vi "Tmp_M simulated main.vi"(8 "Error In":errorcluster, 9 "timeout ms":i32=1000, 10 "Queue to master":T2, 11 "Module queue":T2) -> (0 "Error Out":errorcluster, 1 "Connected":bool=TRUE, 3 "Temperatures":T1[](array[typedef]) {"Time stamp" format="%<%H:%M:%S%2u\n%Y/%m/%d>T"})   [LabVIEW 2021, in "Magnet module.lvlib"]
doc: "Magnet module controls: power supply unit (PSU/SMS) and temperature monitor (TM/LSC218).\nPSU controls mainly: switch heater and ramping of current which runs throught coil.\nTM controls temperature of switch, coil and cryostat.\nMessage for magnet is a cluster that contains: {(enum) Command , (variant) Data}\nFor simplifieing of documentation, the Command is noted as a name of instruction, and Data is represented by a requered datatype (mostly cluster) name.\nCommands:\nInitialize(Magnet Config Constants) - Sugesstion: Load configuration constants from configuration file.\nSet field (Set field{B, R, cr}) - B-field[T], R-ramp[A/s], cr - custom ramp[bool].\nSwitch mode(mode) - to persistant, or to ramping.\nBlackout() - undone functionality of emergency deenergizing.\nUpdate() - Important! This triggers update of data from instruments. Shoud occure in regular intervals as priority message.\nResponses:\nMagnet initialized ();\nTM revision(temperature monitor revision);\nMagnet init error(error);\nSetting field(Set Field{B, R, cr});\nWarning(string);\nSwitching to(mode);\nUpdate error(error);\nTM update(TM sensors);\nPSU update(PSU data);\nMagnet status();"
uses:
  Magnet module.lvlib
  ctl/Cryostat temperature sensors.ctl
  Messenger service/Data types/Module name.ctl
  Messenger service/MessengerLib.lvlib
  submodules/Temperature monitor/Temperature monitor.lvlib
  Messenger service/Data types/Mailbox address.ctl
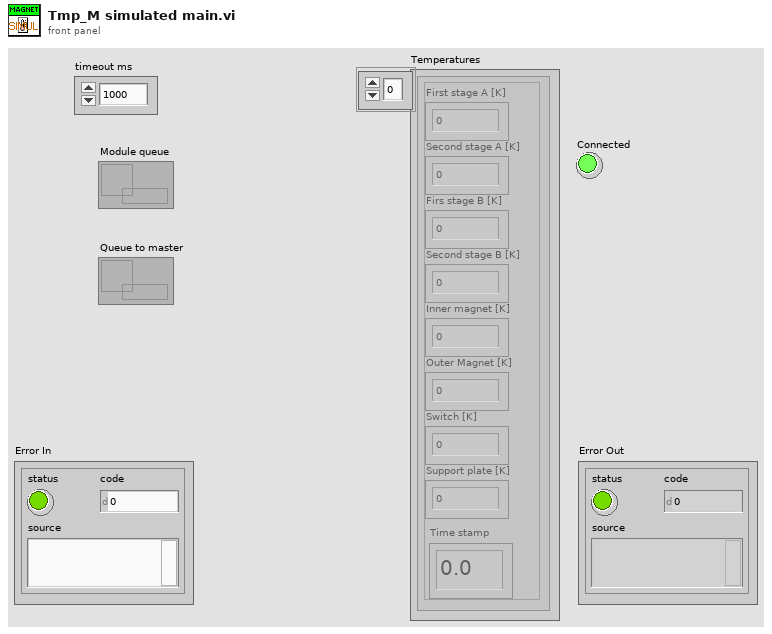
[diagram p1: front panel]
types:
  T1 = typedef "Cryostat temperature sensors.ctl" = cluster{"First stage A [K]":dbl, "Second stage A [K]":dbl, "Firs stage B [K]":dbl, "Second stage B [K]":dbl, "Inner magnet [K]":dbl, "Outer Magnet [K]":dbl, "Switch [K]":dbl, "Support plate [K]":dbl, "Time stamp":dbl}
  T2 = typedef "MessengerLib.lvlib/Mailbox address.ctl" = refnum<queue>
  T3 = typedef "MessengerLib.lvlib/Module name.ctl" = enum16{"Emty", "Magnet", "VTI", "Excitation", "Servo", "Acquisition", "Rotator", "Digitizer", "SMU2450", "Carousel", "Multimeter", "Tmp monitor", "Power monitor"}
  T4 = typedef "Temperature monitor.lvlib/Tmp_M commands.ctl" = enum16{"Ignore", "Log", "Connect", "Set timeout", "Update", "Disconnect", "End"}
  T5 = typedef "Temperature monitor.lvlib/TM Revision.ctl" = cluster{"Instr Serial Number":string, "Instr Driver Revision":string, "Instr Firmware Revision":string, "Instr Model Number":string}
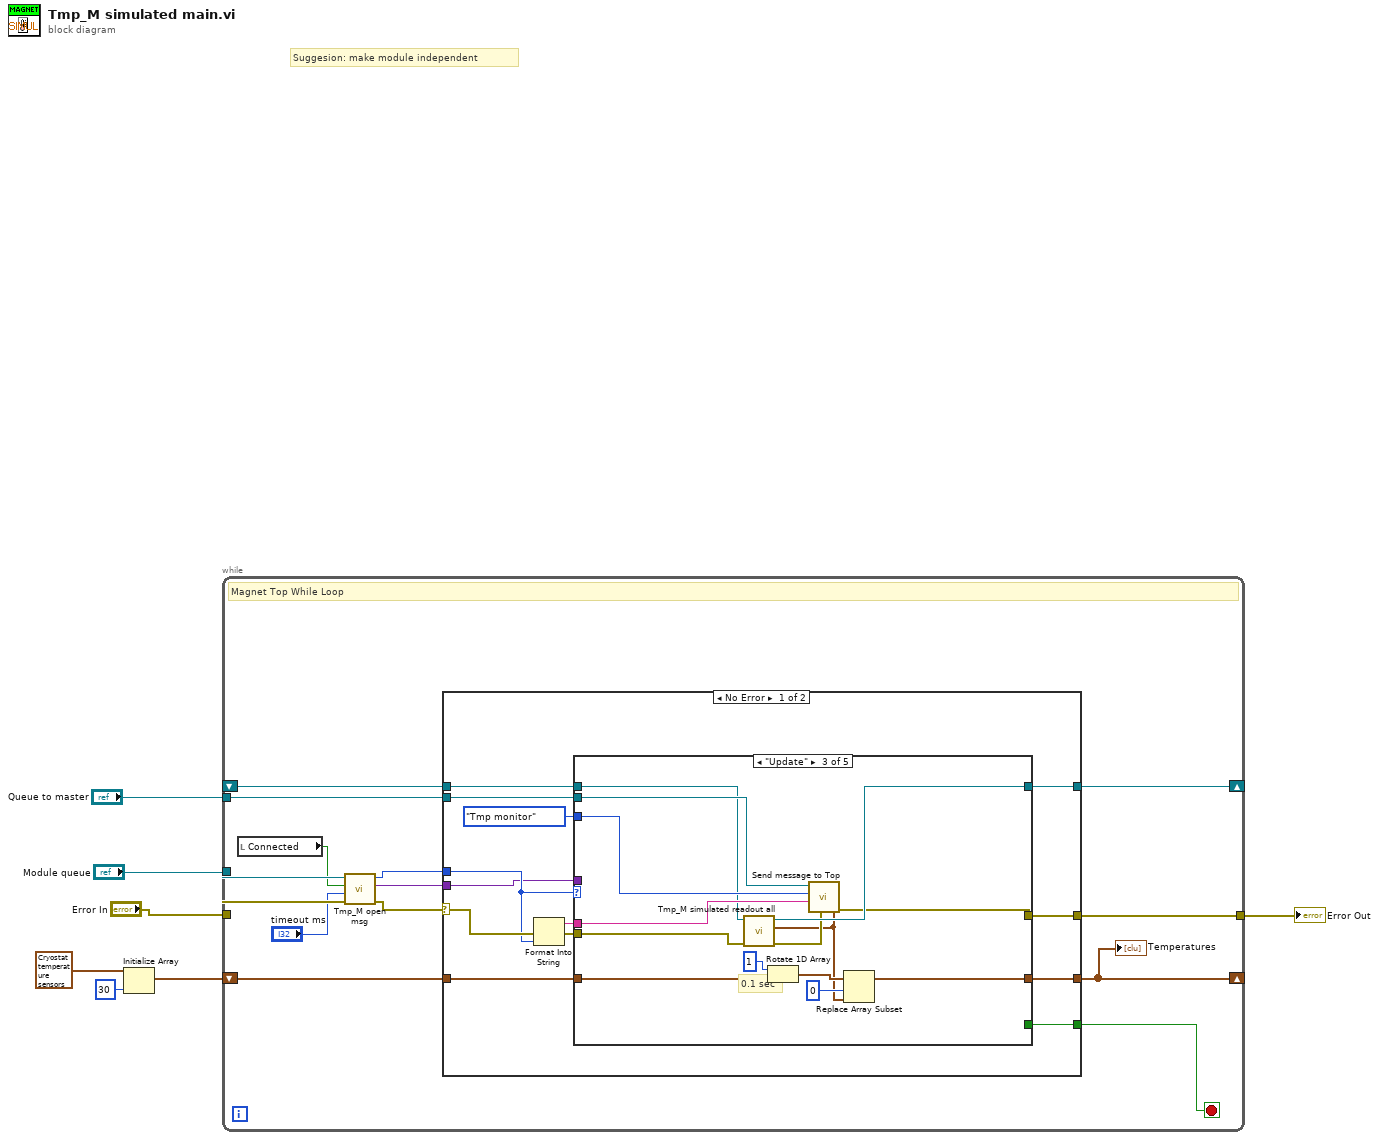
[diagram p0: block diagram]
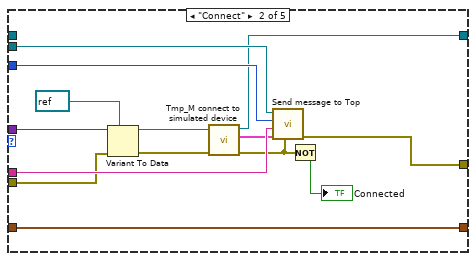
[diagram p3: hidden frame]
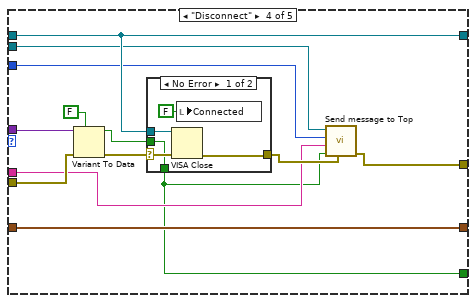
[diagram p4: hidden frame]
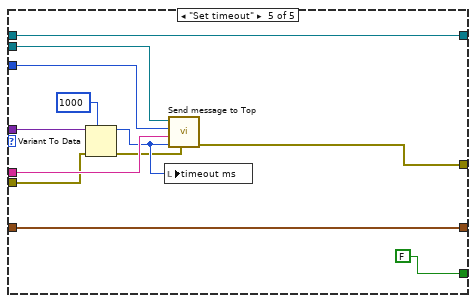
[diagram p6: hidden frame]
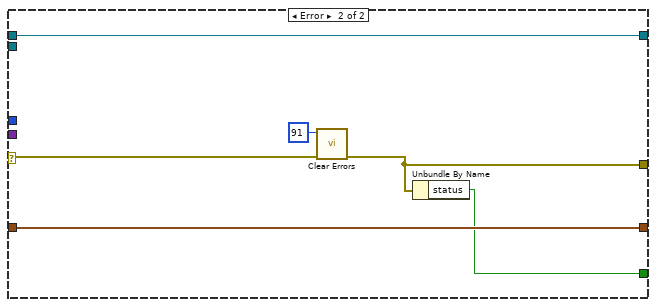
[diagram p7: hidden frame]
diagram:
  # "Suggesion: make module independent"
  n1 = Initialize Array(T1 {"First stage A [K]"=0.0, "Second stage A [K]"=0.0, "Firs stage B [K]"=0.0, "Second stage B [K]"=0.0, "Inner magnet [K]"=0.0, "Outer Magnet [K]"=0.0, "Switch [K]"=0.0, "Support plate [K]"=0.0, "Time stamp"=0.0} ("LSC218 sensors"), 30 ("dimension size")) -> (w5:T1[])
  n2 = while {
    tunnel: "Module queue" -> [w16]
    tunnel: "Queue to master" -> [w21]
    shift-right: [w19] -> _
    shift-left: w5 -> [w20]
    shift-right: [w18] -> _
    shift-left: _ -> [w17]
    tunnel: "Error In" -> [w15]
    tunnel: [w10] -> w1
    stop <- w9 stop-if-true
    # "Magnet Top While Loop"
    n3 = local read "Connected"() -> (w8:bool)
    n4 = call "Tmp_M open msg.vi"("error in (no error)"=w15, "timeout ms (1000)"="timeout ms", "Connected"=w8, "Queue in"=w16) -> ("error out"=w12:errorcluster, "Data"=w11:variant, "Command"=w14:T4)  [unwired: 3 in, 2 out]
    n5 = case shown="No Error" w12 {
      selector: w12 -> [w26 w101]
      tunnel: w21 -> [w34 _]
      tunnel: w14 -> [w25 _]
      tunnel: w20 -> [w33 w102]
      tunnel: [w32 w102] -> w19
      tunnel: [w22 w98] -> w9
      tunnel: [w29 w97] -> w18
      tunnel: w17 -> [w28 w97]
      tunnel: w11 -> [w24 _]
      tunnel: [w23 w99] -> w10
      frame No Error {
        n6 = Format Into String(error in=w26, w25) -> (resulting string=w30:string, error out=w27:errorcluster)  [unwired: 2 in]
        n7 = case shown="\"Update\"" w25 {
          tunnel: w34 -> [_ w51 w61 w70 w95]
          tunnel: w33 -> [w37 w50 w65 w78 w96]
          tunnel: [w37 w50 w64 w78 w96] -> w32
          tunnel: Module_name."Tmp monitor" ("Module") -> [_ w48 w62 w69 w92]
          tunnel: w30 -> [_ w49 w63 w68 w93]
          tunnel: [_ _ _ w66 FALSE] -> w22
          tunnel: [w36 w46 w59 w77 w91] -> w29
          tunnel: w28 -> [w36 _ w60 w77 w91]
          tunnel: w27 -> [w35 w42 w57 w74 w88]
          tunnel: w24 -> [_ w41 _ w75 w89]
          tunnel: [w35 w40 w58 w71 w85] -> w23
          frame "Ignore", Default {
          }
          frame "Connect" {
            n8 = Variant To Data(error in=w42, type=refnum<visa-resource-name> refnum ("LSC218"), Variant=w41) -> (data=w45:refnum<visa-resource-name>, error out=w38:errorcluster)
            n9 = call "Tmp_M connect to simulated device.vi"("error in (no error)"=w38, "VISA Refnum in"=w45) -> ("error out"=w43:errorcluster, "TM Revision"=w47:T5, "VISA Refnum out"=w46:refnum<visa-resource-name>)  [unwired: 7 in]
            n10 = call "Send message to Top.vi"("Error in (no error)"=w43, "Data"=w47, "Response"=w49, "Module"=w48, "Mailbox address in"=w51) -> ("Error out"=w40:errorcluster)  [unwired: 5 in, 1 out]
            n11 = Not(x=w43) -> (.not. x?=→"Connected":bool)
          }
          frame "Update" {
            # "0.1 sec"
            n12 = call "Tmp_M simulated readout all.vi"("error in (no error)"=w57, "VISA Refnum in"=w60) -> ("error out"=w53:errorcluster, "LSC218 sensors"=w52:T1, "VISA Refnum out"=w59:refnum<visa-resource-name>)  [unwired: 7 in]
            n13 = Rotate 1D Array(1:w65, 2:1 ("n")) -> (0:w55:T1[])
            n14 = call "Send message to Top.vi"("Error in (no error)"=w53, "Data"=w52, "Response"=w63, "Module"=w62, "Mailbox address in"=w61) -> ("Error out"=w58:errorcluster)  [unwired: 5 in, 1 out]
            n15 = Replace Array Subset(array=w55, new element=w52, index=0) -> (w64:T1[])
          }
          frame "Disconnect" {
            n16 = Variant To Data(error in=w74, type=FALSE, Variant=w75) -> (data=w67:bool, error out=w73:errorcluster)
            n17 = case shown="No Error" w73 {
              selector: w73 -> [w82 w84]
              tunnel: w77 -> [w83 _]
              tunnel: [w81 w84] -> w72
              tunnel: w67 -> [w79 _]
              tunnel: [w79 _] -> w66
              frame No Error {
                n18 = VISA Close(VISA resource name=w83, error in (no error)=w82) -> (error out=w81:errorcluster)
                n19 = local write "Connected"(FALSE ("Initialized")) -> ()
              }
              frame Error {
              }
            }
            n20 = call "Send message to Top.vi"("Error in (no error)"=w72, "Data"=w66, "Response"=w68, "Module"=w69, "Mailbox address in"=w70) -> ("Error out"=w71:errorcluster)  [unwired: 5 in, 1 out]
          }
          frame "Set timeout" {
            n21 = Variant To Data(error in=w88, type=1000 ("timeout ms"), Variant=w89) -> (data=w87:i32, error out=w86:errorcluster)
            n22 = local write "timeout ms"(w87) -> ()
            n23 = call "Send message to Top.vi"("Error in (no error)"=w86, "Data"=w87, "Response"=w93, "Module"=w92, "Mailbox address in"=w95) -> ("Error out"=w85:errorcluster)  [unwired: 5 in, 1 out]
          }
        }
      }
      frame Error {
        n24 = call <vilib>:"Clear Errors.vi"("error in (no error)"=w101, "specific error code to clear (0: all)"=91) -> ("error out"=w99:errorcluster)  [unwired: 4 in, 1 out]
        n25 = Unbundle By Name(w99) -> ("status"=w98:bool)
      }
    }
    "Temperatures" <- w19
  }
  "Error Out" <- w1
